vi "Aquire CI Encode.vi"() -> ()   [LabVIEW 2017]
panel:
  out "Count":dbl caption="位置"
  out "Direction":string caption="方向"
  out "Speed":dbl caption="速度"
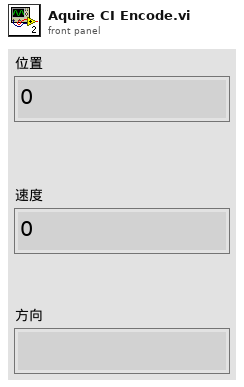
[diagram p1: front panel]
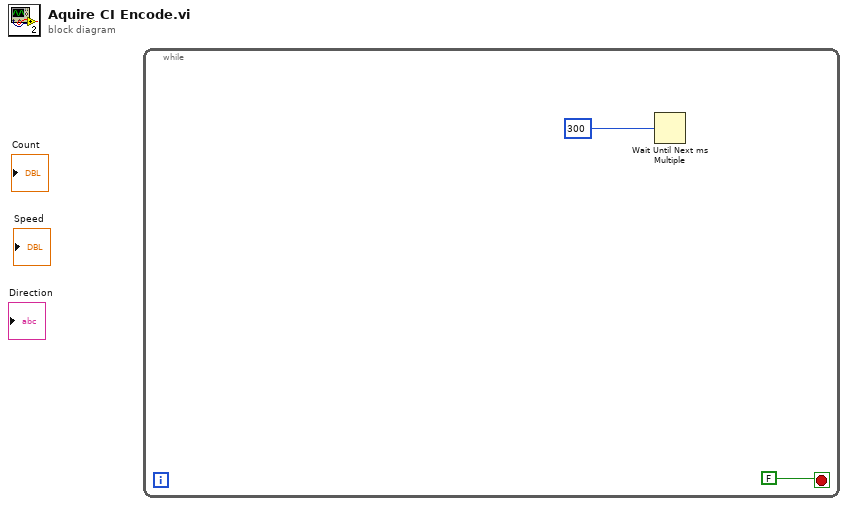
[diagram p0: block diagram]
diagram:
  n1 = while {
    stop <- FALSE stop-if-true
    n2 = Wait Until Next ms Multiple(millisecond multiple=300) -> ()  [unwired: 1 out]
  }
